vi "_write.vi"(8 "Error in (no error)":errorcluster, 10 "Log in":T1 {"Priority" items=["EMERGENCY", "ALERT", "CRITICAL", "ERROR", "WARNING", "NOTICE", "INFO", "DEBUG"]}, 11 "LogWriterStream in":refnum<class "LogWriterStream.lvclass">) -> (0 "Error out":errorcluster, 3 "LogWriterStream out":refnum<class "LogWriterStream.lvclass">)   [LabVIEW 2011, in "LogWriterStream.lvclass"]
uses:
  LogWriterStream.lvclass
  Log/LogCluster.ctl
  Log/PrioritiesRing.ctl
  LogWriterStream.lvclass/LogWriterStream.ctl
  Formatter/LogFormatterInterface/LogFormatterInterface.lvclass
  LogWriterInterface/LogWriterInterface.lvclass
  Log/Log.lvclass
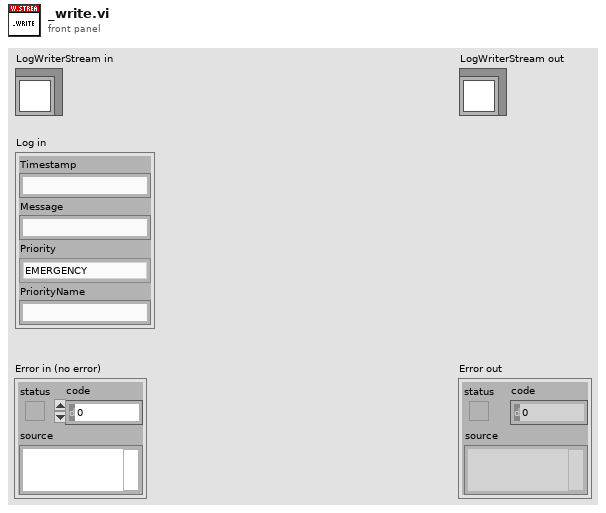
[diagram p1: front panel]
types:
  T1 = typedef "Log.lvclass/LogCluster.ctl" = cluster{"Timestamp":string, "Message":string, "Priority":T2, "PriorityName":string}
  T2 = typedef "Log.lvclass/PrioritiesRing.ctl" = u32
  T3 = enum16{"open", "replace", "create", "open or create", "replace or create", "replace or create with confirmation"}
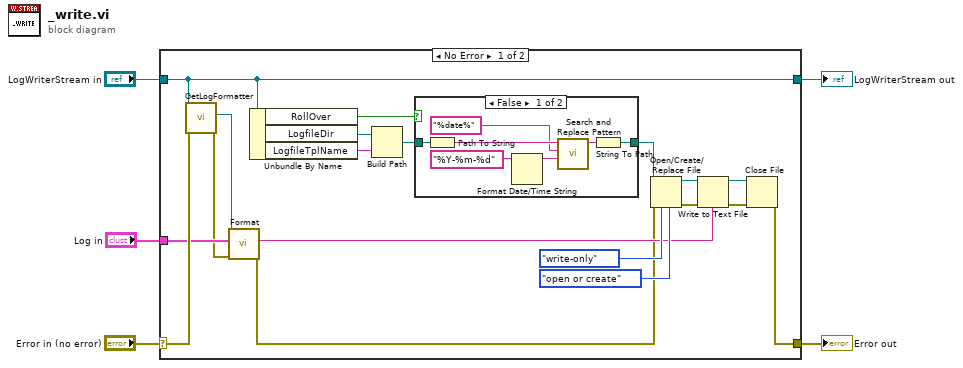
[diagram p0: block diagram]
diagram:
  n1 = case shown="No Error" "Error in (no error)" {
    selector: "Error in (no error)" -> [w24 w34]
    tunnel: [w6 w34] -> w4
    tunnel: [w16 w33] -> w2
    tunnel: "LogWriterStream in" -> [w16 w33]
    tunnel: "Log in" -> [w22 _]
    frame No Error {
      n2 = call "GetLogFormatter.vi"("Error in (no error)"=w24, "LogWriterInterface in"=w16) -> ("Error out"=w20:errorcluster, "LogFormatterInterface out"=w21:refnum<class "LogFormatterInterface.lvclass">)  [unwired: 7 in, 1 out]
      n3 = call-dynamic "Format.vi"("Error in (no error)"=w20, "Log in"=w22, "LogFormatterInterface in"=w21) -> ("Error out"=w7:errorcluster, "Log formatted"=w10:string)  [unwired: 6 in, 1 out]
      n4 = Unbundle By Name(w16) -> ("RollOver"=w23:bool, "LogfileDir"=w19:path, "LogfileTplName"=w18:string)
      n5 = Build Path(base path=w19, name or relative path=w18) -> (appended path=w17:path)
      n6 = case shown="False" w23 {
        tunnel: w17 -> [w31 w32]
        tunnel: [w25 w32] -> w14
        frame False {
          n7 = Path To String(path=w31) -> (string=w30:string)
          n8 = Format Date/Time String(time format string (%c)="%Y-%m-%d") -> (date/time string=w27:string)  [unwired: 2 in]
          n9 = call <vilib>:"Search and Replace Pattern.vi"("string"=w30, "regular expression (\"\")"="%date%" ("regular expression (\"\")"), "replace string (\"\")"=w27) -> ("result string"=w26:string)  [unwired: 2 in, 1 out]
          n10 = String To Path(string=w26) -> (path=w25:path)
        }
        frame True {
        }
      }
      n11 = Open/Create/Replace File(file path (use dialog)=w14, error in=w7, operation (0:open)=T3."open or create", access (0:read/write)=enum16{"read/write", "read-only", "write-only"}."write-only") -> (refnum out=w15:refnum<file>, error out=w11:errorcluster)  [unwired: 2 in, 1 out]
      n12 = Write to Text File(file (use dialog)=w15, text=w10, error in=w11) -> (refnum out=w9:refnum<file>, error out=w8:errorcluster)  [unwired: 1 in, 1 out]
      n13 = Close File(refnum=w9, error in=w8) -> (error out=w6:errorcluster)  [unwired: 1 out]
    }
    frame Error {
    }
  }
  "Error out" <- w4
  "LogWriterStream out" <- w2
